vi "Parse Arguments.vi"(8 "error in (no error)":errorcluster, 10 "Inputs":string[](array[string]), 11 "LUnitCLI In":refnum<class "LUnitCLI.lvclass">) -> (0 "error out":errorcluster, 3 "LUnitCLI Out":refnum<class "LUnitCLI.lvclass">)   [LabVIEW 2020, in "LUnitCLI.lvclass"]
uses:
  LUnitCLI.lvclass
  LUnitCLI.lvclass/LUnitCLI.ctl
  <vilib>/ErrorRing/Error Ring.xnode
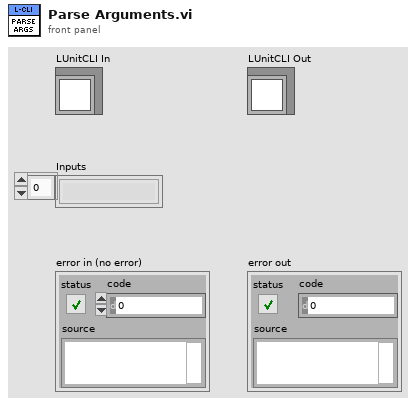
[diagram p1: front panel]
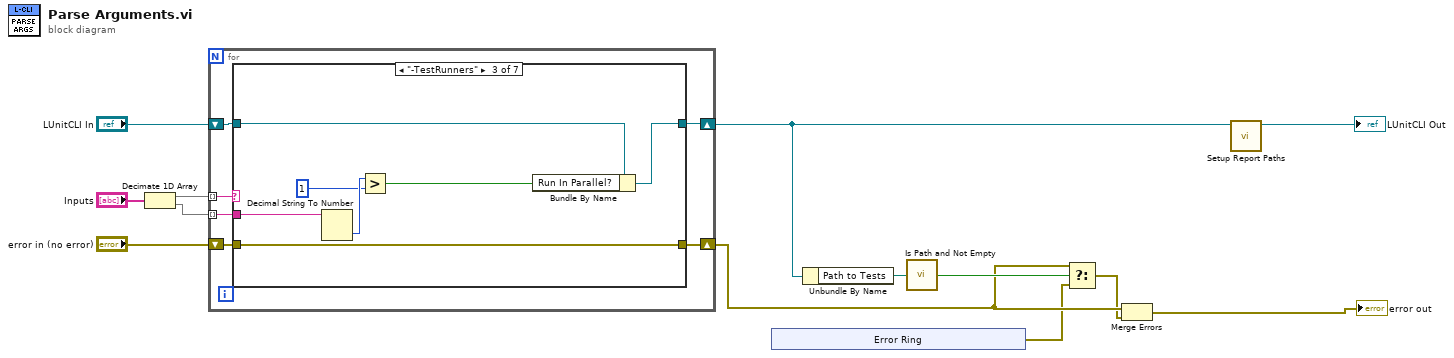
[diagram p0: block diagram]
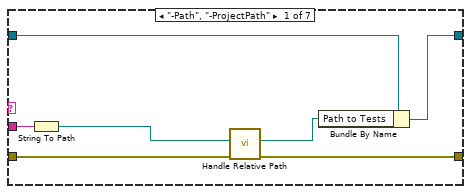
[diagram p2: hidden frame]
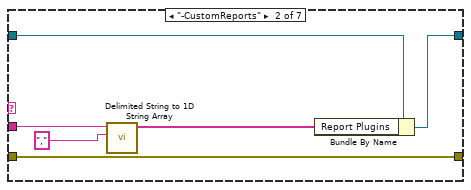
[diagram p3: hidden frame]
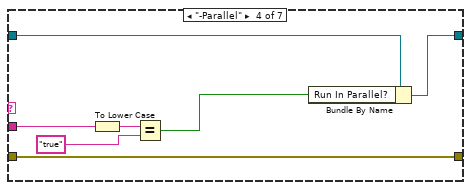
[diagram p4: hidden frame]
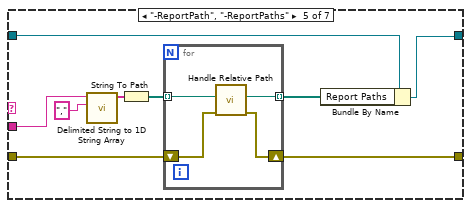
[diagram p5: hidden frame]
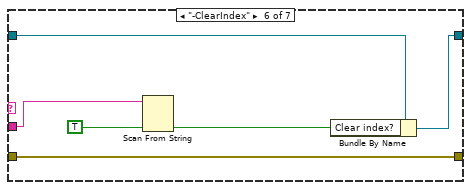
[diagram p6: hidden frame]
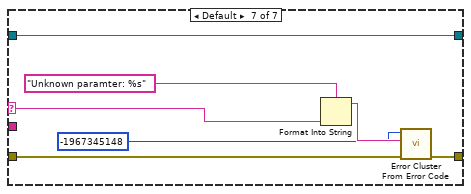
[diagram p7: hidden frame]
diagram:
  n1 = Decimate 1D Array("Inputs") -> (w10:string[], w11:string[])
  n2 = for {
    tunnel: w10 -> [w19] mode=indexing
    tunnel: w11 -> [w18] mode=indexing
    shift-right: [w16] -> w1
    shift-left: "LUnitCLI In" -> [w17]
    shift-right: [w15] -> w5
    shift-left: "error in (no error)" -> [w14]
    n3 = case shown="\"-TestRunners\"" w19 {
      selector: w19 -> [_ _ _ _ _ _ w71]
      tunnel: w18 -> [w25 w27 w36 w43 w47 w62 _]
      tunnel: w17 -> [w20 w32 w39 w46 w51 w65 w66]
      tunnel: [w26 w31 w38 w45 w50 w64 w66] -> w16
      tunnel: [w24 w30 w37 w44 w54 w63 w70] -> w15
      tunnel: w14 -> [w23 w30 w37 w44 w55 w63 w67]
      frame "-Path", "-ProjectPath" {
        n4 = String To Path(string=w25) -> (path=w22:path)
        n5 = call "Handle Relative Path.vi"("error in (no error)"=w23, "Path"=w22) -> ("error out"=w24:errorcluster, "appended path"=w21:path)  [unwired: 8 in]
        n6 = Bundle By Name(cluster=w20, "Path to Tests"=w21) -> (w26:refnum<class "LUnitCLI.lvclass">)
      }
      frame "-CustomReports" {
        n7 = call <vilib>:"Delimited String to 1D String Array.vi"("delimiter"=",", "delimited string"=w27) -> ("string array"=w28:string[])  [unwired: 9 in]
        n8 = Bundle By Name(cluster=w32, "Report Plugins"=w28) -> (w31:refnum<class "LUnitCLI.lvclass">)
      }
      frame "-TestRunners" {
        n9 = Decimal String To Number(string=w36) -> (number=w35:i32)  [unwired: 2 in, 1 out]
        n10 = Greater?(x=w35, y=1) -> (0:w33:bool)
        n11 = Bundle By Name(cluster=w39, "Run In Parallel?"=w33) -> (w38:refnum<class "LUnitCLI.lvclass">)
      }
      frame "-Parallel" {
        n12 = To Lower Case(string=w43) -> (all lower case string=w42:string)
        n13 = Equal?(x=w42, y="true") -> (x = y?=w40:bool)
        n14 = Bundle By Name(cluster=w46, "Run In Parallel?"=w40) -> (w45:refnum<class "LUnitCLI.lvclass">)
      }
      frame "-ReportPath", "-ReportPaths" {
        n15 = call <vilib>:"Delimited String to 1D String Array.vi"("delimiter"=",", "delimited string"=w47) -> ("string array"=w48:string[])  [unwired: 9 in]
        n16 = String To Path(string=w48) -> (path=w53:path[])
        n17 = for {
          tunnel: w53 -> [w57] mode=indexing
          tunnel: [w56] -> w52 mode=indexing
          shift-right: [w58] -> w54
          shift-left: w55 -> [w59]
          n18 = call "Handle Relative Path.vi"("error in (no error)"=w59, "Path"=w57) -> ("error out"=w58:errorcluster, "appended path"=w56:path)  [unwired: 8 in]
        }
        n19 = Bundle By Name(cluster=w51, "Report Paths"=w52) -> (w50:refnum<class "LUnitCLI.lvclass">)
      }
      frame "-ClearIndex" {
        n20 = Scan From String(input string=w62, default 1=TRUE) -> (output 1=w61:bool)  [unwired: 3 in, 3 out]
        n21 = Bundle By Name(cluster=w65, "Clear index?"=w61) -> (w64:refnum<class "LUnitCLI.lvclass">)
      }
      frame Default {
        n22 = Format Into String(format string="Unknown paramter: %s", w71) -> (resulting string=w69:string)  [unwired: 2 in, 1 out]
        n23 = call <vilib>:"Error Cluster From Error Code.vi"("error in (no error)"=w67, "error message (\"\")"=w69, "error code (0)"=-1967345148) -> ("error out"=w70:errorcluster)  [unwired: 6 in]
      }
    }
  }
  n24 = xnode "Error Ring"() -> ("error out"=w4:errorcluster)
  n25 = Unbundle By Name(w1) -> ("Path to Tests"=w8:path)
  n26 = call <vilib>:"Is Path and Not Empty.vi"("path"=w8) -> ("Is Path and Not Empty?"=w6:bool)  [unwired: 4 in]
  n27 = Select(t=w5, s=w6, f=w4) -> (s? t:f=w3:errorcluster)
  n28 = Merge Errors(w5, w3) -> (→"error out":errorcluster)
  n29 = call "Setup Report Paths.vi"("LUnitCLI in"=w1) -> ("LUnitCLI out"=→"LUnitCLI Out":refnum<class "LUnitCLI.lvclass">)  [unwired: 10 in]
